vi "FTW-Endpoint-Payload-Request-Receive.vi"(0 "FTW Endpoint":refnum<class "FTW-Endpoint.lvclass">, 5 "Timeout":i32 format="%dmsec", 11 "error in":errorcluster) -> (4 "FTW Endpoint out":refnum<class "FTW-Endpoint.lvclass">, 6 "Reply Endpoint":refnum<class "FTW-Endpoint.lvclass">, 8 "Payload":T1, 10 "Timed out?":bool, 15 "error out":errorcluster)   [LabVIEW 2013, in "FTW-Endpoint.lvclass"]
uses:
  FTW-Endpoint.lvclass
  Payload/FTW-MessagePayload.ctl
panel:
  # "Inputs"
  # "Outputs"
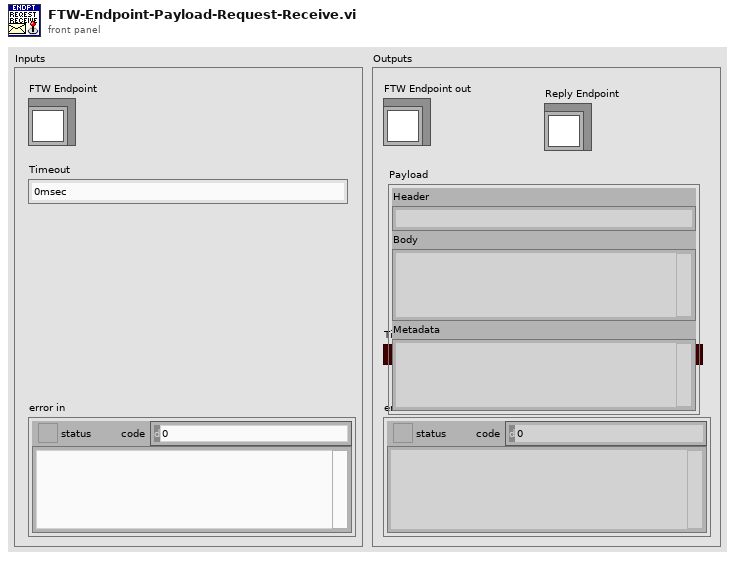
[diagram p1: front panel]
types:
  T1 = typedef "FTW-MessagePayload.ctl" = cluster{"Header":string, "Body":string, "Metadata":string}
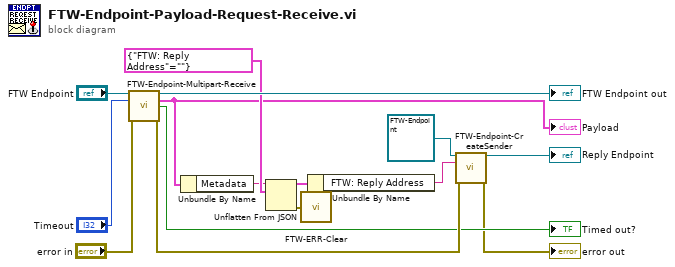
[diagram p0: block diagram]
diagram:
  n1 = call-dynamic "FTW-Endpoint-Multipart-Receive.vi"("FTW Endpoint"="FTW Endpoint", "Timeout"="Timeout", "error in"="error in") -> ("FTW Endpoint out"=→"FTW Endpoint out":refnum<class "FTW-Endpoint.lvclass">, "Message Received"=w2:T1, "Timed out?"=→"Timed out?":bool, "error out"=w15:errorcluster)  [unwired: 9 in]
  "Payload" <- w2
  n2 = Unbundle By Name(w2) -> ("Metadata"=w6:string)
  n3 = Unflatten From JSON(JSON string=w6, type and defaults=cluster{"FTW: Reply Address":string} {"FTW: Reply Address"=""}) -> (value=w7:cluster{"FTW: Reply Address":string}, error out=w8:errorcluster)  [unwired: 5 in]
  n4 = call "FTW-ERR-Clear.vi"("error to snuff"=w8) -> ()  [unwired: 1 out]
  n5 = Unbundle By Name(w7) -> ("FTW: Reply Address"=w5:string)
  n6 = call-dynamic "FTW-Endpoint-CreateSender.vi"("FTW Endpoint"=refnum<class "FTW-Endpoint.lvclass"> refnum, "Endpoint Address"=w5, "error in"=w15) -> ("FTW Endpoint out"=→"Reply Endpoint":refnum<class "FTW-Endpoint.lvclass">, "error out"=→"error out":errorcluster)  [unwired: 11 in]
